vi "Log General Event Helper.vi"(8 "error in (no error)":errorcluster, 9 "Payload":string, 10 "State Info":string, 11 "EventLog in":refnum<class "EventLog.lvclass">) -> (0 "error out":errorcluster, 3 "EventLog out":refnum<class "EventLog.lvclass">)   [LabVIEW 2015, in "Tool Module.lvlib"]
uses:
  Tool Module.lvlib
  QC-X App/Libraries/Event Logger Library/Event Log/EventLog.lvclass
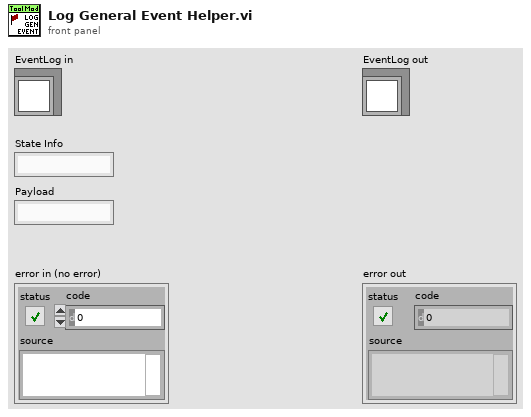
[diagram p1: front panel]
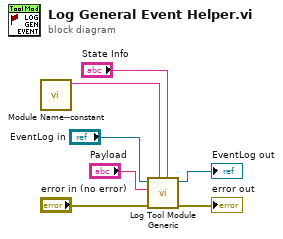
[diagram p0: block diagram]
diagram:
  n1 = call "Module Name--constant.vi"() -> ("Module Name"=w7:string)  [unwired: 11 in]
  n2 = call "Log Tool Module Generic.vi"("State Info"="State Info", "Module Name"=w7, "error in (no error)"="error in (no error)", "Payload"="Payload", "EventLog in"="EventLog in") -> ("error out"=→"error out":errorcluster, "EventLog out"=→"EventLog out":refnum<class "EventLog.lvclass">)  [unwired: 5 in]
